vi "Fault Injection.vi"(4 "settings.<user name>":T2, 8 "unfaulted DO":bool, 11 "state data in":T1) -> (0 "faulted DO":bool)   [LabVIEW 2015, in "Engine Simulation Toolkit.lvlib" / "Digital Pattern Generation.lvlib"]
uses:
  Digital Pattern Generation.lvlib
  Settings.ctl
  state data.ctl
  Engine Simulation Toolkit.lvlib
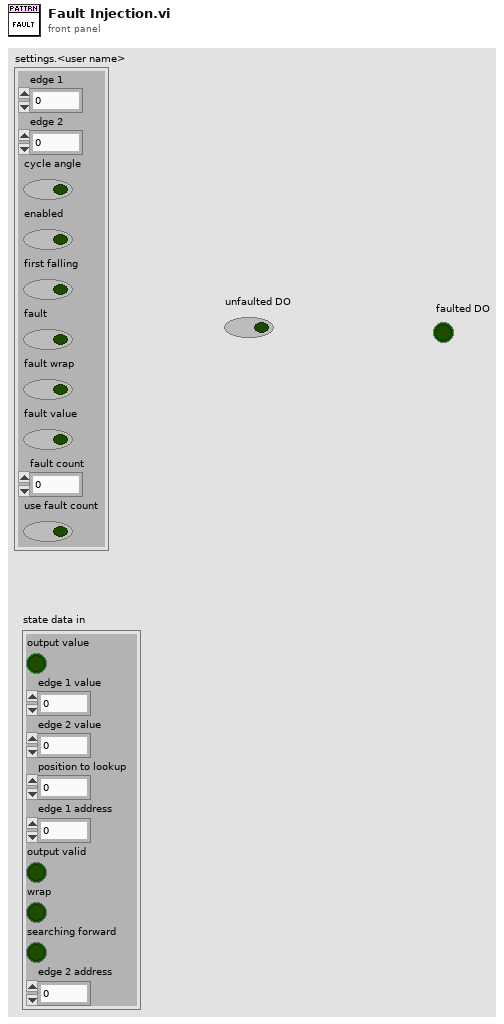
[diagram p1: front panel]
types:
  T1 = typedef "Engine Simulation Toolkit.lvlib/Digital Pattern Generation.lvlib/state data.ctl" = cluster{"output value":bool, "edge 1 value":u16, "edge 2 value":u16, "position to lookup":u16, "edge 1 address":fxp<+,11,11>, "output valid":bool, "wrap":bool, "searching forward":bool, "edge 2 address":fxp<+,11,11>}
  T2 = typedef "Engine Simulation Toolkit.lvlib/Digital Pattern Generation.lvlib/Settings.ctl" = cluster{"edge 1":u16, "edge 2":u16, "cycle angle":bool, "enabled":bool, "first falling":bool, "fault":bool, "fault wrap":bool, "fault value":bool, "fault count":fxp<+,4,4>, "use fault count":bool}
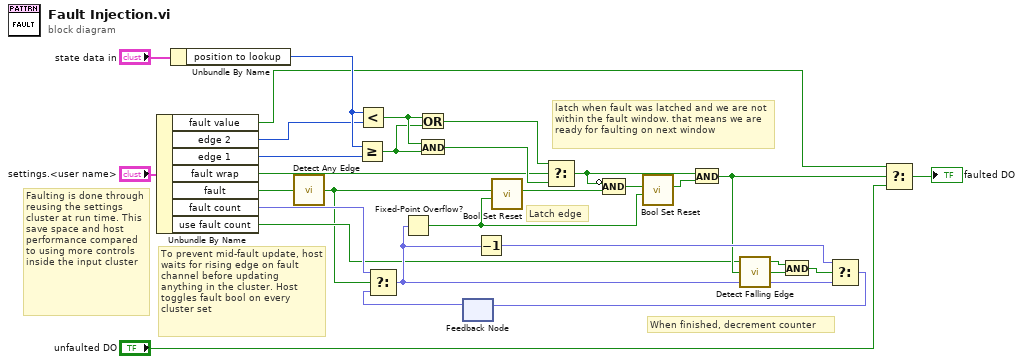
[diagram p0: block diagram]
diagram:
  # "To prevent mid-fault update, host waits for rising edge on fault channel before updating anything in the cluster. Host toggles fault bool on every cluster set"
  # "When finished, decrement counter"
  # "Faulting is done through reusing the settings cluster at run time. This save space and host performance compared to using more controls inside the input cluster"
  # "latch when fault was latched and we are not within the fault window. that means we are ready for faulting on next window"
  # "Latch edge"
  n1 = Unbundle By Name("settings.<user name>") -> ("fault value"=w4:bool, "edge 2"=w21:u16, "edge 1"=w22:u16, "fault wrap"=w5:bool, "fault"=w2:bool, "fault count"=w18:fxp<+,4,4>, "use fault count"=w3:bool)
  n2 = Unbundle By Name("state data in") -> ("position to lookup"=w23:u16)
  n3 = call "Detect Any Edge.vi"("signal"=w2) -> ("edge detected"=w1:bool)  [unwired: 14 in]
  n4 = Greater Or Equal?(x=w23, y=w22) -> (x >= y?=w24:bool)
  n5 = Less?(x=w23, y=w21) -> (x < y?=w25:bool)
  n6 = Or(x=w25, y=w24) -> (x .or. y?=w27:bool)
  n7 = And(x=w25, y=w24) -> (x .and. y?=w26:bool)
  n8 = feedback #1() -> (w17:fxp<+,4,4>)  [unwired: 1 in]
  n9 = Select(t=w18, s=w1, f=w17) -> (s? t:f=w9:fxp<+,4,4>)
  n10 = Fixed-Point Overflow?(1:w9) -> (0:w8:bool)
  n11 = Decrement(x=w9) -> (x-1=w16:fxp<+,4,4>)
  n12 = call "Bool Set Reset.vi"("clear"=w8, "set"=w1) -> ("out"=w12:bool)  [unwired: 9 in]
  n13 = Select(t=w27, s=w5, f=w26) -> (s? t:f=w13:bool)
  n14 = Compound Arithmetic op=AND(invert w13, w12) -> (w11:bool)
  n15 = call "Bool Set Reset.vi"("clear"=w8, "set"=w11) -> ("out"=w14:bool)  [unwired: 9 in]
  n16 = And(x=w13, y=w14) -> (x .and. y?=w10:bool)
  n17 = call "Detect Falling Edge.vi"("signal"=w10) -> ("edge detected"=w7:bool)  [unwired: 14 in]
  n18 = And(x=w3, y=w7) -> (x .and. y?=w6:bool)
  n19 = Select(t=w16, s=w6, f=w9) -> (s? t:f=w15:fxp<+,4,4>)
  n20 = feedback-in #1(w15) -> ()
  n21 = Select(t=w4, s=w10, f="unfaulted DO") -> (s? t:f=→"faulted DO":bool)
